vi "GetBankingTransactions.vi"(8 "error in (no error)":errorcluster, 10 "WhichMonth":refnum<class "WhichMonth.lvclass">, 11 "Database in":refnum<class "Account History.lvclass">) -> (0 "error out":errorcluster, 2 "Banking Transactions out":refnum<class "BankingTransactionList.lvclass">, 3 "Database out":refnum<class "Account History.lvclass">)   [LabVIEW 2020, in "Account History.lvclass"]
uses:
  Account History.lvclass
  WhichMonth/WhichMonth.lvclass
  Banking Statement/BankingTransactionList.lvclass
  C:/GitRepos/Filthy-Lucre-Budgetizer/source/support/classes/Statement/TransactionList.lvclass
  Banking Record/BankingTransaction.lvclass
  C:/GitRepos/Filthy-Lucre-Budgetizer/source/support/classes/Transaction/Transaction.lvclass
  Statement/TransactionList.lvclass
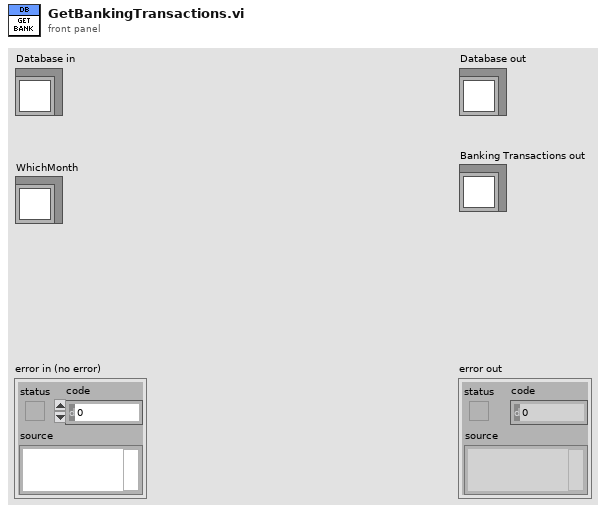
[diagram p1: front panel]
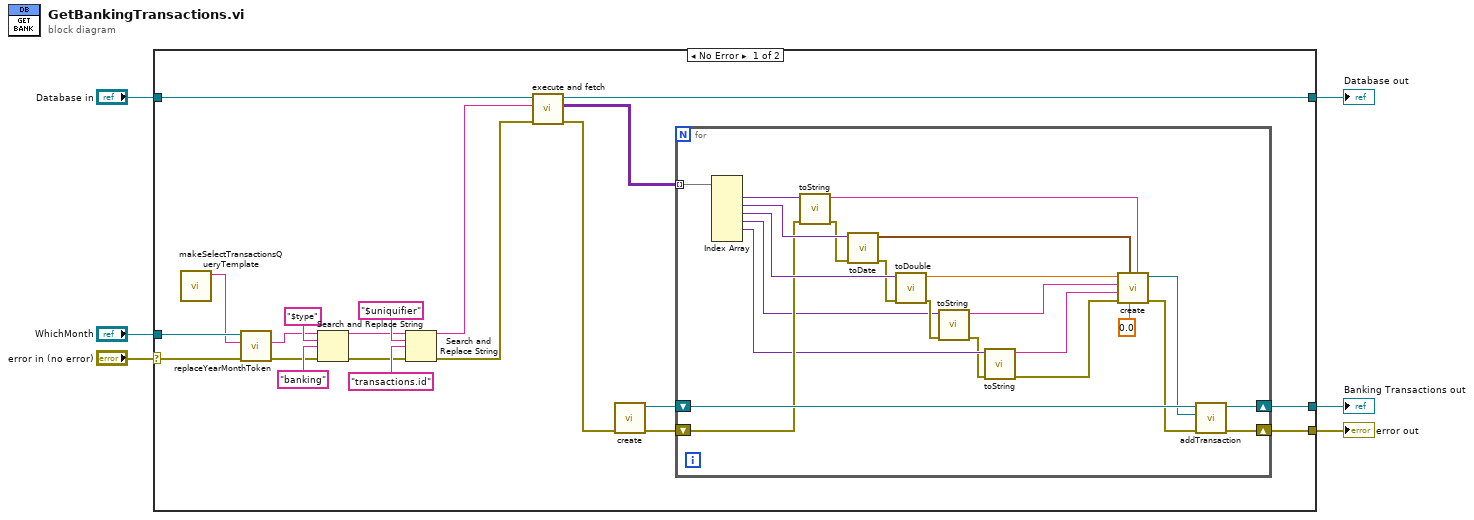
[diagram p0: block diagram]
diagram:
  n1 = case shown="No Error" "error in (no error)" {
    selector: "error in (no error)" -> [w23 w52]
    tunnel: [w21 w52] -> w3
    tunnel: [w26 w51] -> w5
    tunnel: "Database in" -> [w27 w51]
    tunnel: "WhichMonth" -> [w24 _]
    tunnel: [w20 _] -> w1
    frame No Error {
      n2 = call "makeSelectTransactionsQueryTemplate.vi"() -> ("SELECT Query"=w22:string)  [unwired: 11 in]
      n3 = call "replaceYearMonthToken.vi"("error in (no error)"=w23, "Query In"=w22, "WhichMonth in"=w24) -> ("error out"=w14:errorcluster, "Query Out"=w13:string)  [unwired: 6 in, 1 out]
      n4 = Search and Replace String(input string=w13, search string="$type", replace string="banking", error in=w14) -> (result string=w10:string, error out=w9:errorcluster)  [unwired: 4 in, 2 out]
      n5 = Search and Replace String(input string=w10, search string="$uniquifier", replace string="transactions.id", error in=w9) -> (result string=w7:string, error out=w8:errorcluster)  [unwired: 4 in, 2 out]
      n6 = call "execute and fetch.vi"("error in (no error)"=w8, "SQL query"=w7, "Database in"=w27) -> ("error out"=w17:errorcluster, "recordset data"=w25:variant[][], "Database out"=w26:refnum<class "Account History.lvclass">)  [unwired: 6 in]
      n7 = call "create.vi"("error in (no error)"=w17) -> ("error out"=w18:errorcluster, "Banking Transactions out"=w19:refnum<class "BankingTransactionList.lvclass">)  [unwired: 9 in]
      n8 = for {
        shift-right: [w49] -> w20
        shift-left: w19 -> [w50]
        shift-right: [w48] -> w21
        shift-left: w18 -> [w35]
        tunnel: w25 -> [w45] mode=indexing
        n9 = Index Array(array=w45) -> (element #1=w44:variant, element #2=w42:variant, element #3=w40:variant, element #4=w31:variant, element #5=w30:variant)  [unwired: 6 in, 1 out]
        n10 = call "toString.vi"("error in (no error)"=w35, "Variant"=w44) -> ("error out"=w34:errorcluster, "String"=w43:string)  [unwired: 8 in]
        n11 = call "toDate.vi"("error in (no error)"=w34, "Variant"=w42) -> ("error out"=w33:errorcluster, "time stamp"=w41:timestamp)  [unwired: 8 in]
        n12 = call "toDouble.vi"("error in (no error)"=w33, "Value"=w40) -> ("error out"=w32:errorcluster, "type"=w39:dbl)  [unwired: 8 in]
        n13 = call "toString.vi"("error in (no error)"=w32, "Variant"=w31) -> ("error out"=w29:errorcluster, "String"=w37:string)  [unwired: 8 in]
        n14 = call "toString.vi"("error in (no error)"=w29, "Variant"=w30) -> ("error out"=w28:errorcluster, "String"=w36:string)  [unwired: 8 in]
        n15 = call "create.vi"("Reference"=w43, "Balance"=0.0, "Date"=w41, "error in (no error)"=w28, "Category"=w36, "Description"=w37, "Amount"=w39) -> ("error out"=w46:errorcluster, "Banking Transaction out"=w47:refnum<class "BankingTransaction.lvclass">)  [unwired: 3 in]
        n16 = call "addTransaction.vi"("error in (no error)"=w46, "Transaction.lvclass"=w47, "TransactionList in"=w50) -> ("error out"=w48:errorcluster, "TransactionList out"=w49:refnum<class "BankingTransactionList.lvclass">)  [unwired: 7 in]
      }
    }
    frame Error {
    }
  }
  "error out" <- w3
  "Database out" <- w5
  "Banking Transactions out" <- w1
